vi "fg_display_multiplier.vi"(8 "error in (no error)":errorcluster, 10 "multiplier":i32, 11 "n_data in":i32) -> (0 "error out":errorcluster, 3 "n_data out":i32)   [LabVIEW 2015, in "lv-graph.lvlib"]
uses:
  lv-graph.lvlib
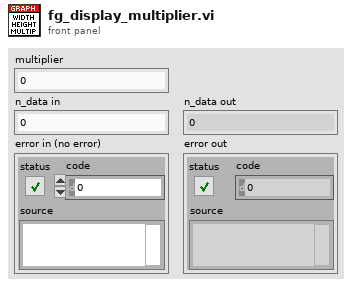
[diagram p1: front panel]
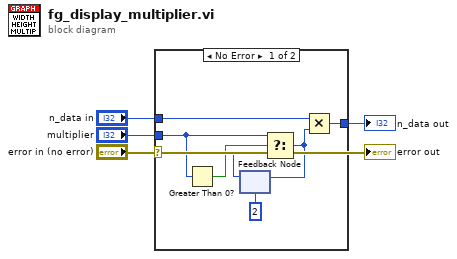
[diagram p0: block diagram]
diagram:
  n1 = case shown="No Error" "error in (no error)" {
    tunnel: "n_data in" -> [w11 _]
    tunnel: [w10 _] -> w3
    tunnel: "multiplier" -> [w9 _]
    frame No Error {
      n2 = Greater Than 0?(x=w9) -> (x > 0?=w7:bool)
      n3 = feedback #1(u32 2 ("f")) -> (w5:u32)
      n4 = Select(t=w9, s=w7, f=w5) -> (s? t:f=w8:u32)
      n5 = feedback-in #1(w8) -> ()
      n6 = Multiply(x=w11, y=w8) -> (x*y=w10:u32)
    }
    frame Error {
    }
  }
  "n_data out" <- w3
  "error out" <- "error in (no error)"
